vi "Log.vi"(8 "error in (no error)":errorcluster, 10 "UUID":string, 11 "CubeLogger in":refnum<class "CubeLogger.lvclass">) -> (0 "error out":errorcluster, 1 "Repeat?":bool, 2 "UUID to re-enqueue":string, 3 "CubeLogger out":refnum<class "CubeLogger.lvclass">, 4 "Finished?":bool, 6 "Ready?":bool)   [LabVIEW 2018, in "CubeLogger.lvclass"]
uses:
  CubeLogger.lvclass
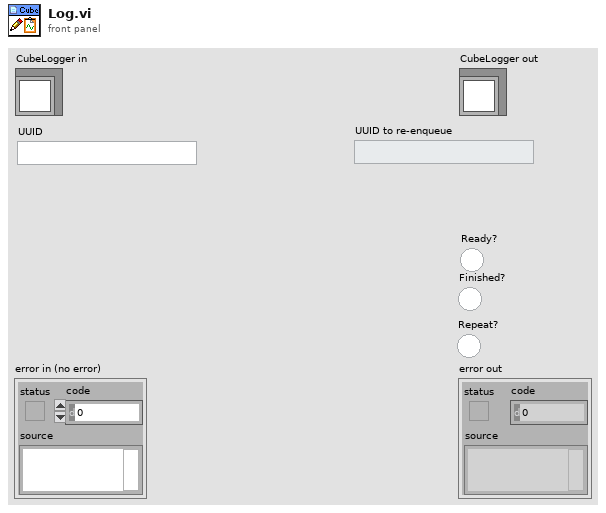
[diagram p1: front panel]
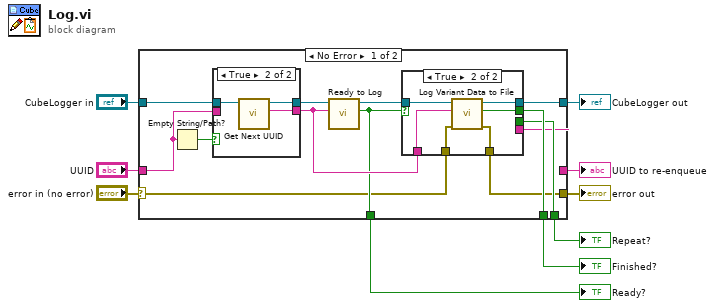
[diagram p0: block diagram]
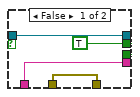
[diagram p2: hidden frame]
diagram:
  n1 = case shown="No Error" "error in (no error)" {
    selector: "error in (no error)" -> [w11 w39]
    tunnel: [w10 w39] -> w8
    tunnel: [w16 w38] -> w6
    tunnel: "CubeLogger in" -> [w21 w38]
    tunnel: "UUID" -> [w20 _]
    tunnel: [w15 _] -> w4
    tunnel: [w14 _] -> w3
    tunnel: [w13 _] -> w2
    tunnel: [w12 _] -> w1
    frame No Error {
      n2 = Empty String/Path?(string/path=w20) -> (empty?=w22:bool)
      n3 = case shown="True" w22 {
        tunnel: w21 -> [w34 w37]
        tunnel: [w33 w36] -> w17
        tunnel: [w34 w35] -> w19
        tunnel: w20 -> [w33 _]
        frame False {
        }
        frame True {
          n4 = call "Get Next UUID.vi"("CubeLogger in"=w37) -> ("UUID"=w36:string, "CubeLogger out"=w35:refnum<class "CubeLogger.lvclass">)  [unwired: 8 in, 1 out]
        }
      }
      n5 = call "Ready to Log.vi"("UUID"=w17, "CubeLogger in"=w19) -> ("Ready?"=w15:bool, "CubeLogger out"=w18:refnum<class "CubeLogger.lvclass">)  [unwired: 7 in, 1 out]
      n6 = case shown="True" w15 {
        tunnel: w18 -> [w26 w32]
        tunnel: w17 -> [w24 w31]
        tunnel: [w26 w30] -> w16
        tunnel: [_ w29] -> w14
        tunnel: [TRUE ("Repeat?") _] -> w13
        tunnel: [w24 _] -> w12
        tunnel: w11 -> [w23 w28]
        tunnel: [w23 w27] -> w10
        frame False {
        }
        frame True {
          n7 = call-dynamic "Log Variant Data to File.vi"("error in (no error)"=w28, "UUID"=w31, "CubeLogger in"=w32) -> ("error out"=w27:errorcluster, "Finished?"=w29:bool, "CubeLogger out"=w30:refnum<class "CubeLogger.lvclass">)  [unwired: 6 in]
        }
      }
    }
    frame Error {
    }
  }
  "error out" <- w8
  "CubeLogger out" <- w6
  "Ready?" <- w4
  "Finished?" <- w3
  "Repeat?" <- w2
  "UUID to re-enqueue" <- w1
